vi "Demo Grab.vi"() -> ()   [LabVIEW 2010]
uses:
  <vilib>/Utility/error.llb/DialogType.ctl
panel:
  out "picture":picture caption="Image"
  in  "Timeout Frame":i32=2000
  out "Index Loop":i32
  out "Index Image":i32
  out "Image":T1(plugin-control)
  in  "?":bool
  out "Height":i32
  out "Width":i32
  out "FPS":dbl
  in  "Source":string="http://217.211.159.251:8080/axis-cgi/mjpg/video.cgi?resolution=640x480"
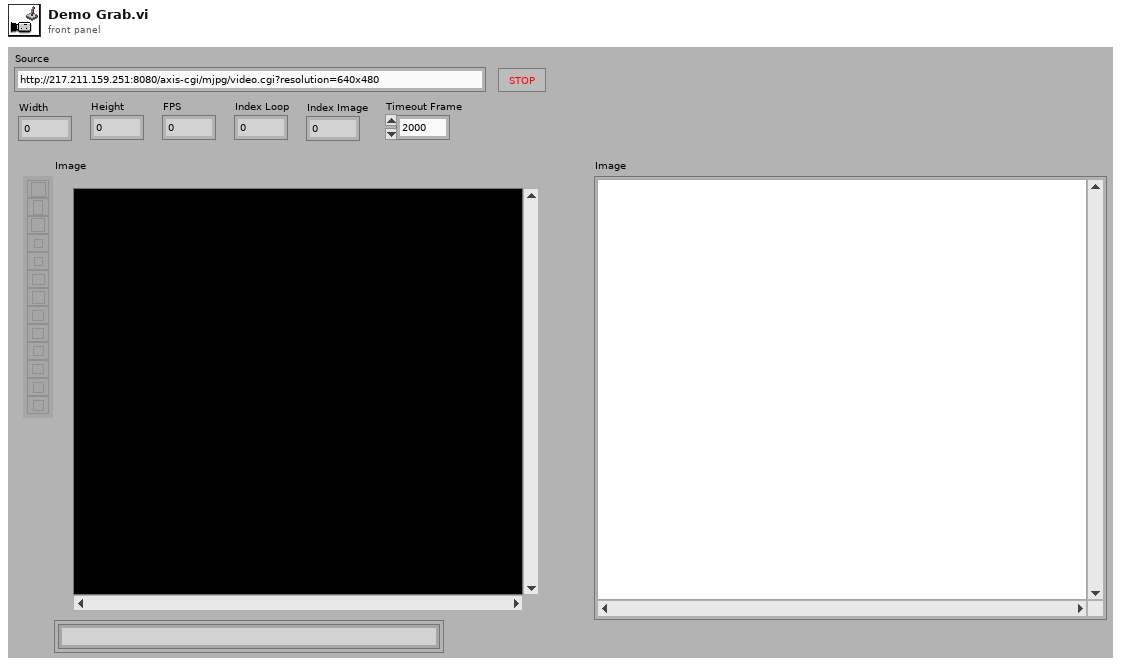
[diagram p1: front panel]
types:
  T1 = typedef "IMAQ Image.ctl" = refnum<image>
  T2 = typedef "Image Type" = u32
  T3 = typedef "DialogType.ctl" = u16
  T4 = typedef "imagedata.ctl" = cluster{"image type":i32, "image depth":i32, "image":u8[], "mask":u8[], "colors":u32[], "Rectangle":cluster{"left":i16, "top":i16, "right":i16, "bottom":i16}}
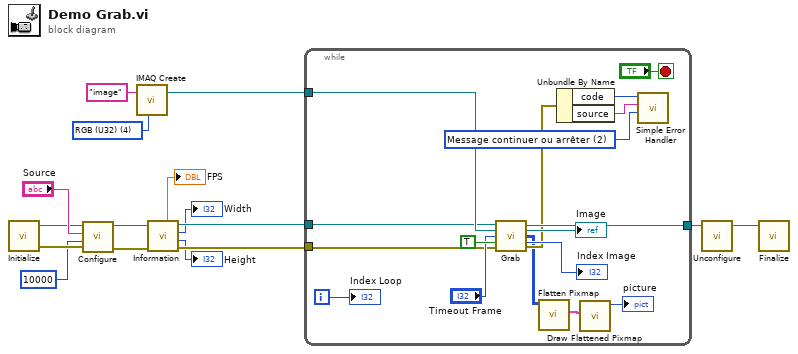
[diagram p0: block diagram]
diagram:
  w12 = T2 4 items=["Grayscale (U8)", "Grayscale (I16)", "Grayscale (SGL)", "Complex (CSG)", "RGB (U32)", "HSL (U32)", "RGB (U64)", "Grayscale (U16)"] ("Image Type")
  n1 = call "Initialize.vi"() -> ("error out"=w11:errorcluster, "ref out"=w4:refnum<k7>)  [unwired: 4 in]
  n2 = call "Configure.vi"("error in"=w11, "timeout"=10000 ("Timeout"), "source"="Source", "ref in"=w4) -> ("error out"=w8:errorcluster, "ref out"=w7:refnum<k7>)  [unwired: 2 in]
  n3 = call "IMAQ Create"("Image Name"="image", "Image Type"=w12) -> ("New Image"=w14:T1)  [unwired: 3 in, 1 out]
  n4 = call "Information.vi"("error in"=w8, "ref in"=w7) -> ("error out"=w15:errorcluster, "height"=→"Height":i32, "width"=→"Width":i32, "ref out"=w16:refnum<k7>, "fps"=→"FPS":dbl)  [unwired: 5 in]
  n5 = while {
    tunnel: w16 -> [w21]
    tunnel: [w33] -> w6
    tunnel: w14 -> [w29]
    tunnel: w15 -> [w20]
    i -> [w30]
    stop <- "?" stop-if-true
    w23 = T3 2 items=["pas de dialogue", "Message OK", "Message continuer ou arrêter", "Message OK + mises en garde", "Arrêter/Continuer + mises en garde"] ("type of dialog (OK msg:1)")
    n6 = call "Grab.vi"("ref in"=w21, "image in"=w29, "Timeout"="Timeout Frame", "wait"=TRUE ("Wait"), "error in"=w20) -> ("ref out"=w33:refnum<k7>, "image out"=→"Image":T1, "pixel"=w17:u32[][], "index"=→"Index Image":i32, "error out"=w26:errorcluster)  [unwired: 6 in]
    n7 = call <vilib>:"Flatten Pixmap.vi"("24-bit pixmap"=w17) -> ("image data"=w19:T4)  [unwired: 10 in]
    n8 = Unbundle By Name(w26) -> ("code"=w24:i32, "source"=w25:string)
    n9 = call <vilib>:"Draw Flattened Pixmap.vi"("image data"=w19) -> ("new picture"=→"picture":picture)  [unwired: 8 in]
    n10 = call <vilib>:"Simple Error Handler.vi"("error code (no error:0)"=w24, "error source (\" \")"=w25, "type of dialog (OK msg:1)"=w23) -> ()  [unwired: 2 in, 5 out]
    "Index Loop" <- w30
  }
  n11 = call "Unconfigure.vi"("ref in"=w6) -> ("ref out"=w5:refnum<k7>)  [unwired: 3 in, 1 out]
  n12 = call "Finalize.vi"("ref in"=w5) -> ()  [unwired: 4 in, 1 out]
